vi "create_log_string.vi"(8 "source":string, 9 "thread":string, 10 "Code":i32) -> (3 "log string":string)   [LabVIEW 2019, in "Log.lvlib" / "Log.lvclass"]
uses:
  Log.lvclass
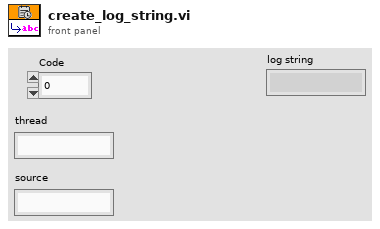
[diagram p1: front panel]
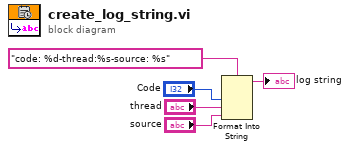
[diagram p0: block diagram]
diagram:
  n1 = Format Into String(format string="code: %d-thread:%s-source: %s" ("格式字符串"), "Code", "thread", "source") -> (resulting string=→"log string":string)  [unwired: 2 in, 1 out]
